vi "Get Tag Location.vi"(10 "tag info":dbl[][](array[numeric]), 11 "tag ID":i32) -> (2 "angle":dbl, 3 "field locations (ft)":cluster{"X":dbl, "Y":dbl})   [LabVIEW 2023]
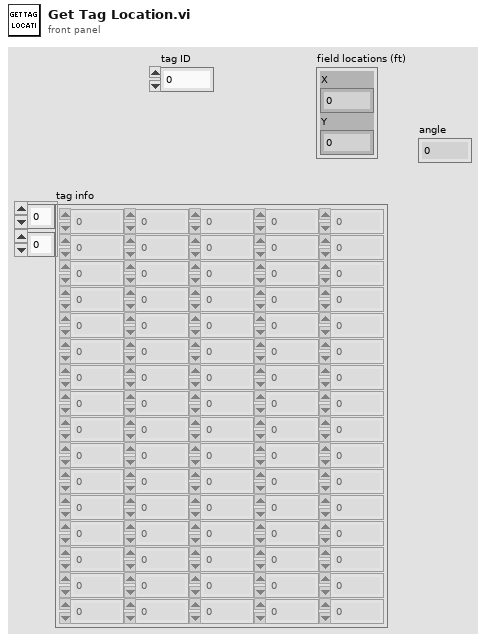
[diagram p1: front panel]
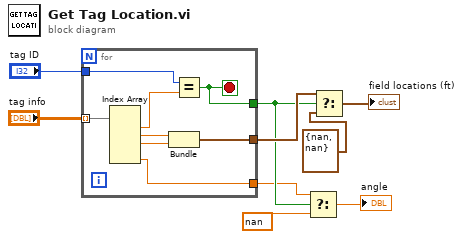
[diagram p0: block diagram]
diagram:
  n1 = for {
    tunnel: "tag info" -> [w15] mode=indexing
    tunnel: [w11] -> w6
    tunnel: "tag ID" -> [w17]
    tunnel: [w16] -> w4
    tunnel: [w10] -> w3
    stop <- w16 stop-if-true
    n2 = Index Array(array=w15) -> (element #1=w14:dbl, element #2=w13:dbl, element #3=w12:dbl, element #5=w10:dbl)  [unwired: 5 in, 1 out]
    n3 = Bundle(w13, w12) -> (w11:cluster{dbl, dbl})  [unwired: 1 in]
    n4 = Equal?(x=w17, y=w14) -> (x = y?=w16:bool)
  }
  n5 = Select(t=w3, s=w4, f=nan) -> (s? t:f=→"angle":dbl)
  n6 = Select(t=w6, s=w4, f=cluster{"X":dbl, "Y":dbl} {"X"=nan, "Y"=nan}) -> (s? t:f=→"field locations (ft)":cluster{"X":dbl, "Y":dbl})
